vi "获取操作日志 (子VI).vi"(11 "table输入":string(combo)) -> ()   [LabVIEW 2016]
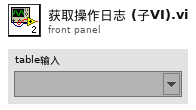
[diagram p1: front panel]
types:
  T1 = enum16{"CODMn", "PH", "氨氮", "总氮", "总磷", "CODCr", "电导率", "水温", "DO", "浊度", "叶绿素", "藻密度"}
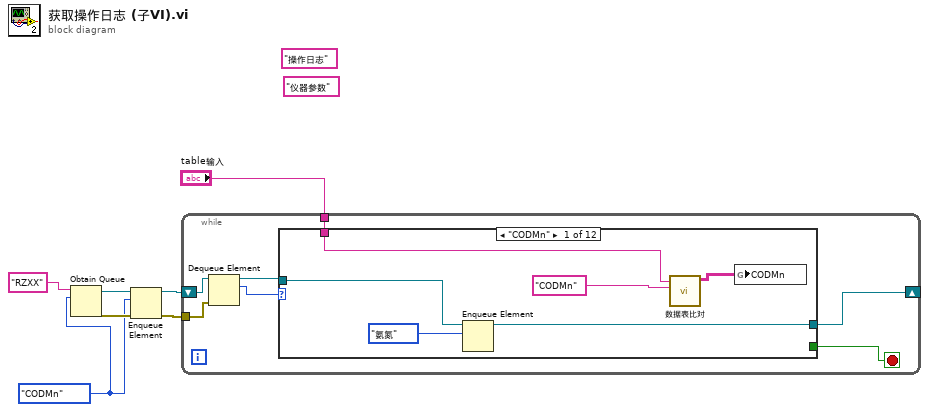
[diagram p0: block diagram]
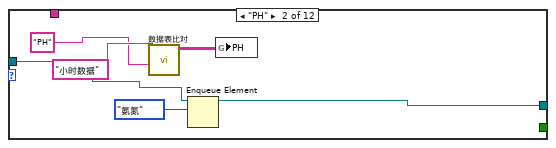
[diagram p2: hidden frame]
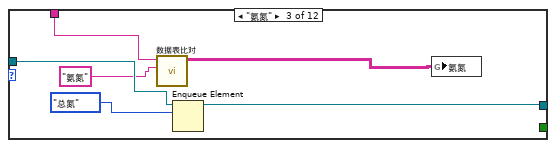
[diagram p3: hidden frame]
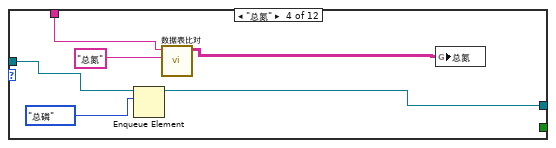
[diagram p4: hidden frame]
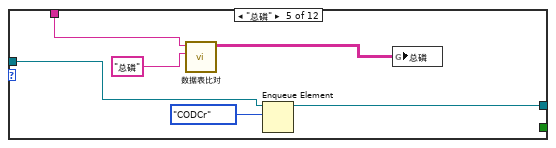
[diagram p5: hidden frame]
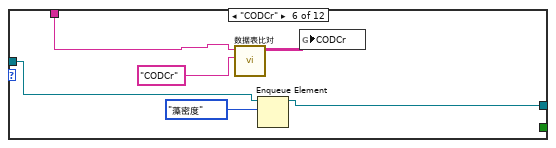
[diagram p6: hidden frame]
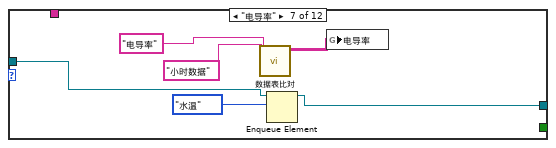
[diagram p7: hidden frame]
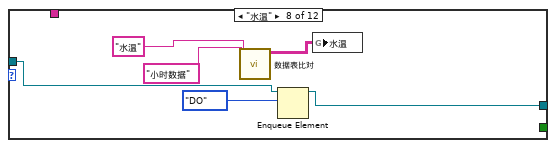
[diagram p8: hidden frame]
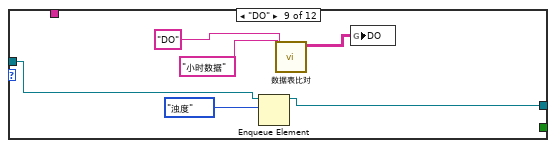
[diagram p9: hidden frame]
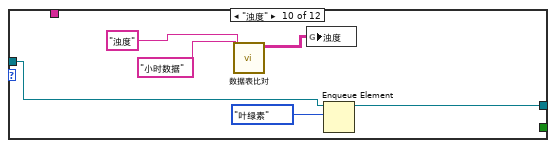
[diagram p10: hidden frame]
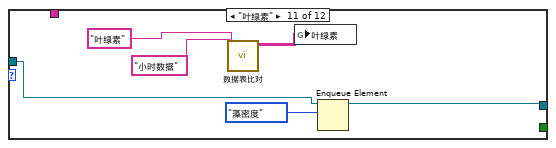
[diagram p11: hidden frame]
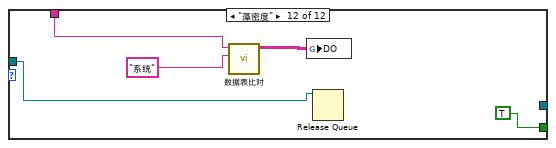
[diagram p12: hidden frame]
diagram:
  (unwired) "仪器参数" ("新元素/子数组")
  (unwired) "操作日志" ("新元素/子数组")
  w2 = T1."CODMn"
  n1 = Obtain Queue(name (unnamed)="RZXX" ("名称（未命名）"), element data type=w2) -> (queue out=w6:refnum<queue>, error out=w3:errorcluster)  [unwired: 3 in, 1 out]
  n2 = Enqueue Element(queue=w6, element=w2, error in (no error)=w3) -> (queue out=w5:refnum<queue>, error out=w4:errorcluster)  [unwired: 1 in, 1 out]
  n3 = while {
    shift-right: [w12] -> _
    shift-left: w5 -> [w14]
    tunnel: w4 -> [w11]
    tunnel: "table输入" -> [w8]
    stop <- w9 stop-if-true
    n4 = Dequeue Element(queue=w14, error in (no error)=w11) -> (queue out=w13:refnum<queue>, element=w10:T1)  [unwired: 1 in, 2 out]
    n5 = case shown="\"CODMn\"" w10 {
      tunnel: w13 -> [w20 w26 w31 w38 w43 w48 w52 w58 w64 w70 w76 w84]
      tunnel: [w19 w25 w32 w37 w42 w47 w51 w57 w63 w69 w75 _] -> w12
      tunnel: [_ _ _ _ _ _ _ _ _ _ _ TRUE] -> w9
      tunnel: w8 -> [w15 _ w27 w33 w39 w45 _ _ _ _ _ w81]
      frame "CODMn" {
        n6 = Enqueue Element(queue=w20, element=T1."氨氮") -> (queue out=w19:refnum<queue>)  [unwired: 2 in, 2 out]
        n7 = call "数据表比对.vi"("仪器日志参数"="CODMn" ("元素"), "table输入"=w15) -> ("待发送数据"=w17:string[][])  [unwired: 6 in, 3 out]
        n8 = global write "全局 所有参数.vi" "CODMn"(w17) -> ()
      }
      frame "PH" {
        n9 = call "数据表比对.vi"("查询元素输入"="PH" ("元素"), "table输入"="小时数据" ("新元素/子数组")) -> ("待发送数据"=w22:string[][])  [unwired: 6 in, 3 out]
        n10 = Enqueue Element(queue=w26, element=T1."氨氮") -> (queue out=w25:refnum<queue>)  [unwired: 2 in, 2 out]
        n11 = global write "全局 所有参数.vi" "PH"(w22) -> ()
      }
      frame "氨氮" {
        n12 = call "数据表比对.vi"("仪器日志参数"="氨氮" ("元素"), "table输入"=w27) -> ("待发送数据"=w29:string[][])  [unwired: 6 in, 3 out]
        n13 = Enqueue Element(queue=w31, element=T1."总氮") -> (queue out=w32:refnum<queue>)  [unwired: 2 in, 2 out]
        n14 = global write "全局 所有参数.vi" "氨氮"(w29) -> ()
      }
      frame "总氮" {
        n15 = Enqueue Element(queue=w38, element=T1."总磷") -> (queue out=w37:refnum<queue>)  [unwired: 2 in, 2 out]
        n16 = call "数据表比对.vi"("仪器日志参数"="总氮" ("元素"), "table输入"=w33) -> ("待发送数据"=w35:string[][])  [unwired: 6 in, 3 out]
        n17 = global write "全局 所有参数.vi" "总氮"(w35) -> ()
      }
      frame "总磷" {
        n18 = call "数据表比对.vi"("仪器日志参数"="总磷" ("元素"), "table输入"=w39) -> ("待发送数据"=w41:string[][])  [unwired: 6 in, 3 out]
        n19 = Enqueue Element(queue=w43, element=T1."CODCr") -> (queue out=w42:refnum<queue>)  [unwired: 2 in, 2 out]
        n20 = global write "全局 所有参数.vi" "总磷"(w41) -> ()
      }
      frame "CODCr" {
        n21 = call "数据表比对.vi"("仪器日志参数"="CODCr" ("元素"), "table输入"=w45) -> ("待发送数据"=w50:string[][])  [unwired: 6 in, 3 out]
        n22 = Enqueue Element(queue=w48, element=T1."藻密度") -> (queue out=w47:refnum<queue>)  [unwired: 2 in, 2 out]
        n23 = global write "全局 所有参数.vi" "CODCr"(w50) -> ()
      }
      frame "电导率" {
        n24 = call "数据表比对.vi"("查询元素输入"="电导率" ("元素"), "table输入"="小时数据" ("新元素/子数组")) -> ("待发送数据"=w54:string[][])  [unwired: 6 in, 3 out]
        n25 = Enqueue Element(queue=w52, element=T1."水温") -> (queue out=w51:refnum<queue>)  [unwired: 2 in, 2 out]
        n26 = global write "全局 所有参数.vi" "电导率"(w54) -> ()
      }
      frame "水温" {
        n27 = call "数据表比对.vi"("查询元素输入"="水温" ("元素"), "table输入"="小时数据" ("新元素/子数组")) -> ("待发送数据"=w60:string[][])  [unwired: 6 in, 3 out]
        n28 = Enqueue Element(queue=w58, element=T1."DO") -> (queue out=w57:refnum<queue>)  [unwired: 2 in, 2 out]
        n29 = global write "全局 所有参数.vi" "水温"(w60) -> ()
      }
      frame "DO" {
        n30 = Enqueue Element(queue=w64, element=T1."浊度") -> (queue out=w63:refnum<queue>)  [unwired: 2 in, 2 out]
        n31 = call "数据表比对.vi"("查询元素输入"="DO" ("元素"), "table输入"="小时数据" ("新元素/子数组")) -> ("待发送数据"=w66:string[][])  [unwired: 6 in, 3 out]
        n32 = global write "全局 所有参数.vi" "DO"(w66) -> ()
      }
      frame "浊度" {
        n33 = call "数据表比对.vi"("查询元素输入"="浊度" ("元素"), "table输入"="小时数据" ("新元素/子数组")) -> ("待发送数据"=w71:string[][])  [unwired: 6 in, 3 out]
        n34 = global write "全局 所有参数.vi" "浊度"(w71) -> ()
        n35 = Enqueue Element(queue=w70, element=T1."叶绿素") -> (queue out=w69:refnum<queue>)  [unwired: 2 in, 2 out]
      }
      frame "叶绿素" {
        n36 = call "数据表比对.vi"("查询元素输入"="叶绿素" ("元素"), "table输入"="小时数据" ("新元素/子数组")) -> ("待发送数据"=w77:string[][])  [unwired: 6 in, 3 out]
        n37 = global write "全局 所有参数.vi" "叶绿素"(w77) -> ()
        n38 = Enqueue Element(queue=w76, element=T1."藻密度") -> (queue out=w75:refnum<queue>)  [unwired: 2 in, 2 out]
      }
      frame "藻密度" {
        n39 = call "数据表比对.vi"("仪器日志参数"="系统" ("元素"), "table输入"=w81) -> ("待发送数据"=w85:string[][])  [unwired: 6 in, 3 out]
        n40 = global write "全局 所有参数.vi" "DO"(w85) -> ()
        n41 = Release Queue(queue=w84) -> ()  [unwired: 2 in, 3 out]
      }
    }
  }
